vi "On Idle.vi"(8 "error in (no error)":errorcluster, 11 "Thing in":refnum<class "Server.lvclass">) -> (0 "error out":errorcluster, 3 "Thing out":refnum<class "Server.lvclass">)   [LabVIEW 2023]
uses:
  Server.lvclass
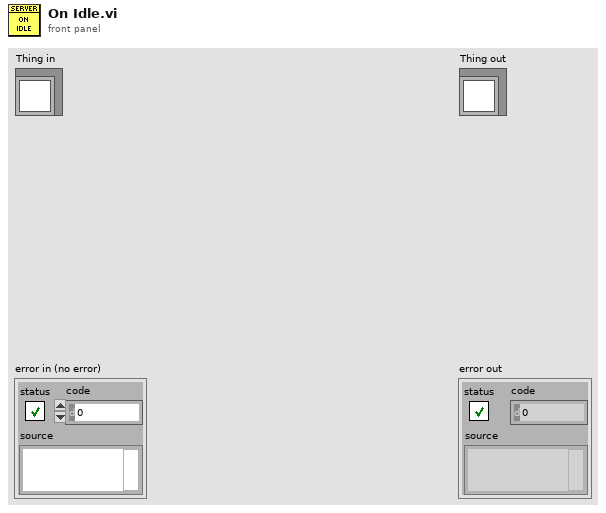
[diagram p1: front panel]
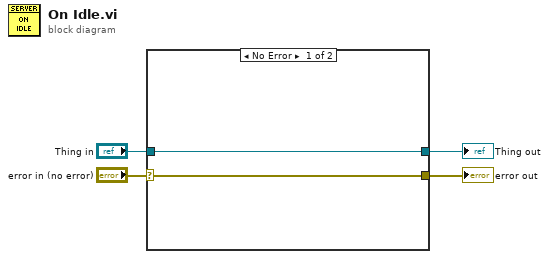
[diagram p0: block diagram]
diagram:
  n1 = case shown="No Error" "error in (no error)" {
    selector: "error in (no error)" -> [w5 w8]
    tunnel: [w5 w8] -> w3
    tunnel: [w6 w7] -> w1
    tunnel: "Thing in" -> [w6 w7]
    frame No Error {
    }
    frame Error {
    }
  }
  "error out" <- w3
  "Thing out" <- w1
